vi "Set Position.vi"(1 "Position":dbl) -> ()   [LabVIEW 2013]
uses:
  PPMS Global.vi
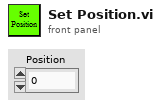
[diagram p1: front panel]
types:
  T1 = enum16{"0", "1", "2", "3", "4", "5", "6", "7", "8", "9", "10", "11", "12", "13", "14"}
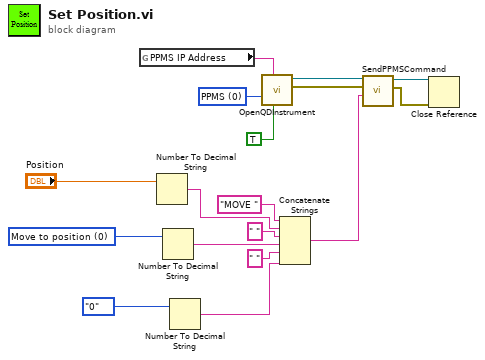
[diagram p0: block diagram]
diagram:
  w7 = 0 items=["PPMS", "VersaLab", "DynaCool", "SVSM"] ("Instrument\nType")
  w14 = u16 0 items=["Move to position", "Move to limit", "Redefine current position", ""] ("Mode")
  n1 = global read "PPMS Global.vi" "PPMS IP Address"() -> (w6:string)
  n2 = Number To Decimal String(number="Position") -> (decimal integer string=w16:string)  [unwired: 1 in]
  n3 = Number To Decimal String(number=w14) -> (decimal integer string=w13:string)  [unwired: 1 in]
  n4 = Number To Decimal String(number=T1."0" ("Slow down code\ndefault = 0")) -> (decimal integer string=w10:string)  [unwired: 1 in]
  n5 = call "OpenQDInstrument.vi"("Remote"=TRUE, "IP Address"=w6, "Instrument Type"=w7) -> ("error out"=w3:errorcluster, "Instrument Ref"=w4:refnum<k24>)  [unwired: 5 in]
  n6 = Concatenate Strings("MOVE " ("string"), w16, " " ("string"), w13, " " ("string"), w10) -> (w9:string)
  n7 = call "SendPPMSCommand.vi"("PpmsCommand"=w9, "error in (no error)"=w3, "Instrument Ref In"=w4) -> ("error out"=w1:errorcluster, "Instrument Ref Out"=w2:refnum<k24>)  [unwired: 4 in, 3 out]
  n8 = Close Reference(reference=w2, error in (no error)=w1) -> ()  [unwired: 1 out]
